vi "SetChannelHW.vi"(8 "error in (no error)":errorcluster, 11 "BME_DG_Base in":refnum<class "BME_DG_Base.lvclass">) -> (0 "error out":errorcluster, 3 "BME_DG_Base out":refnum<class "BME_DG_Base.lvclass">)   [LabVIEW 2009, in "POLARIS BME DG.lvlib" / "BME_DG_Base.lvclass"]
uses:
  BME_DG_Base.lvclass
  BME_DG_Base.lvclass/BME_DG_Base.ctl
  BME_DG_Chnl/BME_DG_Chnl.lvclass
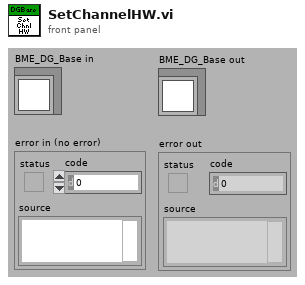
[diagram p1: front panel]
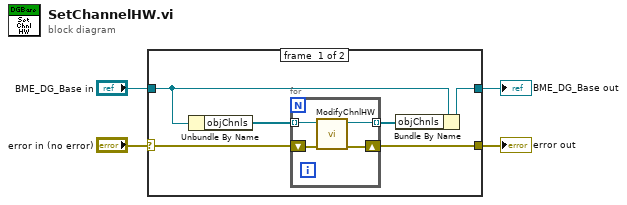
[diagram p0: block diagram]
diagram:
  n1 = case shown="No Error" "error in (no error)" {
    selector: "error in (no error)" -> [w6 w16]
    tunnel: [w5 w16] -> w3
    tunnel: [w8 w15] -> w1
    tunnel: "BME_DG_Base in" -> [w10 w15]
    frame #0 {
      n2 = Unbundle By Name(w10) -> ("objChnls"=w9:refnum<class "BME_DG_Chnl.lvclass">[])
      n3 = for {
        tunnel: w9 -> [w14] mode=indexing
        tunnel: [w13] -> w7 mode=indexing
        shift-right: [w11] -> w5
        shift-left: w6 -> [w12]
        n4 = call-dynamic "ModifyChnlHW.vi"("error in (no error)"=w12, "BME_DG_Chnl in"=w14) -> ("error out"=w11:errorcluster, "BME_DG_Chnl out"=w13:refnum<class "BME_DG_Chnl.lvclass">)  [unwired: 8 in]
      }
      n5 = Bundle By Name(cluster=w10, "objChnls"=w7) -> (w8:refnum<class "BME_DG_Base.lvclass">)
    }
    frame #1 {
    }
  }
  "error out" <- w3
  "BME_DG_Base out" <- w1
